vi "Archiver.vi"() -> ()   [LabVIEW 2016]
uses:
  Archiver.Action.ctl
  tools/CitTemplate/citTemplate.errData.ctl
  tools/EventLog/EventLog.EventSource.ctl
panel:
  out "Folder":string
  out "_loop":i32(ring)=4
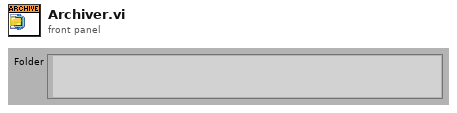
[diagram p1: front panel]
types:
  T1 = typedef "citTemplate.errData.ctl" = cluster{"ts":timestamp, "src":T2, "instance":i32, "action":string, "error":errorcluster, "unconfirmed":bool}
  T2 = typedef "EventLog.EventSource.ctl" = enum16{"All", "Gui", "Ref", "File", "Arch", "Seq", "CPX", "DB", "Laser", "Scan.P", "Scan.O"}
  T3 = typedef "Archiver.Action.ctl" = enum32{"idle", "constructor", "destructor", "--- Archiver ---"}
  T4 = typedef "citTemplate.notifierHandle.ctl" = refnum<notifier>
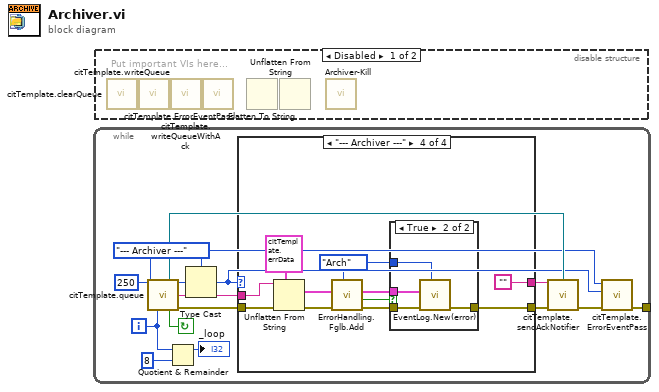
[diagram p0: block diagram]
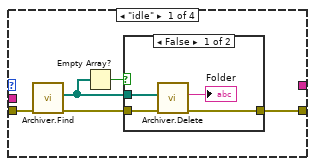
[diagram p3: hidden frame]
diagram:
  n1 = while {
    tunnel: [w2] -> _
    i -> [w4]
    stop <- w11 continue-if-true
    w8 = Archiver.Action."--- Archiver ---" ("Action")
    n2 = call "citTemplate.queue.vi"("ms timeout (250 ms)"=250, "event enum"=w8, "iteration (-1)"=w4) -> ("notifierHandle out"=w10:T4, "event out"=w14:u32, "(flatten) data out"=w13:string, "continue"=w11:bool, "error out"=w12:errorcluster)  [unwired: 2 in, 6 out]
    n3 = Quotient & Remainder(x=w4, y=8) -> (x-y*floor(x/y)=→"_loop":i32)  [unwired: 1 out]
    n4 = Type Cast(type=w8, x=w14) -> (*(type *) &x=w3:T3)
    n5 = case shown="\"--- Archiver ---\"" w3 {
      tunnel: w13 -> [_ _ _ w35]
      tunnel: w12 -> [w19 w25 w26 w34]
      tunnel: [_ _ _ ""] -> w9
      tunnel: [w17 w25 w26 w27] -> w7
      frame "idle" {
        n6 = call "Archiver.Find.vi"("error in"=w19) -> ("error out"=w18:errorcluster, "files to remove"=w15:path[])  [unwired: 9 in]
        n7 = Empty Array?(array=w15) -> (empty?=w16:bool)
        n8 = case shown="False" w16 {
          tunnel: w18 -> [w23 w24]
          tunnel: [w22 w24] -> w17
          tunnel: w15 -> [w21 _]
          frame False {
            n9 = call "Archiver.Delete.vi"("error in"=w23, "files to remove"=w21) -> ("error out"=w22:errorcluster, "last delete element"=→"Folder":string)  [unwired: 8 in]
          }
          frame True {
          }
        }
      }
      frame "constructor" {
      }
      frame "destructor" {
      }
      frame "--- Archiver ---" {
        w28 = EventLog.EventSource."Arch" ("Event source")
        n10 = Unflatten From String(type=T1 {"ts"=timestamp(0 s since 1904-01-01), "src"=enum."All", "instance"=0, "action"="", "error"={"status"=FALSE, "code"=0, "source"=""}, "unconfirmed"=FALSE} ("ErrData"), binary string=w35, error in (no error)=w34) -> (value=w29:T1, error out=w30:errorcluster)  [unwired: 3 out]
        n11 = call "ErrorHandling.Fglb.Add.vi"("Event source"=w28, "error in (no error)"=w30, "Error in"=w29) -> ("error out"=w32:errorcluster, "changed?"=w31:bool)  [unwired: 7 in]
        n12 = case shown="True" w31 {
          tunnel: [w37 w41] -> w27
          tunnel: w29 -> [_ w40]
          tunnel: w32 -> [w37 w39]
          tunnel: w28 -> [_ w38]
          frame False {
          }
          frame True {
            n13 = call "EventLog.New(error).vi"("Source (All)"=w38, "error in"=w39, "ErrData"=w40) -> ("error out"=w41:errorcluster)  [unwired: 8 in]
          }
        }
      }
    }
    n14 = call "citTemplate.sendAckNotifier.vi"("notification data"=w9, "notifierHandle in"=w10, "error in"=w7) -> ()  [unwired: 13 out]
    n15 = call "citTemplate.ErrorEventPass.vi"("error in"=w7, "action of error"=w3, "event in"=w8) -> ("error out"=w2:errorcluster)  [unwired: 2 in, 6 out]
  }
  n16 = disable-structure shown="Disabled" {
    frame Disabled {
      # "Put important VIs here..."
      n17 = call "citTemplate.clearQueue.vi"() -> ()  [unwired: 14 in, 2 out]
      n18 = call "citTemplate.writeQueue.vi"() -> ()  [unwired: 15 in, 1 out]
      n19 = call "citTemplate.writeQueueWithAck.vi"() -> ()  [unwired: 13 in, 3 out]
      n20 = call "citTemplate.ErrorEventPass.vi"() -> ()  [unwired: 11 in, 1 out]
      n21 = Flatten To String() -> ()  [unwired: 4 in, 3 out]
      n22 = Unflatten From String() -> ()  [unwired: 5 in, 3 out]
      n23 = call "Archiver-Kill.vi"() -> ()  [unwired: 11 in, 1 out]
    }
    frame Enabled {
    }
  }
